vi "Convert Cmd Name to Response Name.vi"(11 "cmd name":string) -> (3 "response name":string)   [LabVIEW 2021, in "AudioGenUtility.lvlib"]
uses:
  AudioGenUtility.lvlib
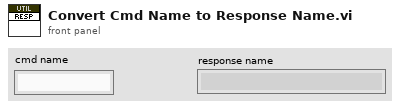
[diagram p1: front panel]
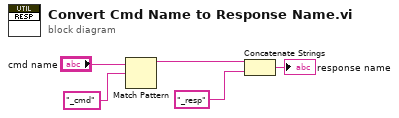
[diagram p0: block diagram]
diagram:
  n1 = Match Pattern(string="cmd name", regular expression="_cmd") -> (before substring=w2:string)  [unwired: 1 in, 3 out]
  n2 = Concatenate Strings(w2, "_resp" ("string")) -> (→"response name":string)
